vi "local.Reserve.vi"(0 "SLSC Local in":refnum<class "SLSC Interface.lvclass">, 5 "devices":refnum<k21>="$DefaultDevices", 7 "reservation access (Read/Write)":i32(ring)=3 items=["Read Only"=1, "Read/Write"=3], 9 "reservation group":string, 11 "error in (no error)":errorcluster) -> (4 "SLSC Local out":refnum<class "SLSC Interface.lvclass">, 15 "error out":errorcluster)   [LabVIEW 2016, in "SLSC Interface.lvclass"]
uses:
  SLSC Interface Class/SLSC Interface.lvclass
  SLSC Interface Class/Read session.vi
  SLSC Interface Class/Write session.vi
  <vilib>/SLSC/SLSC.lvlib
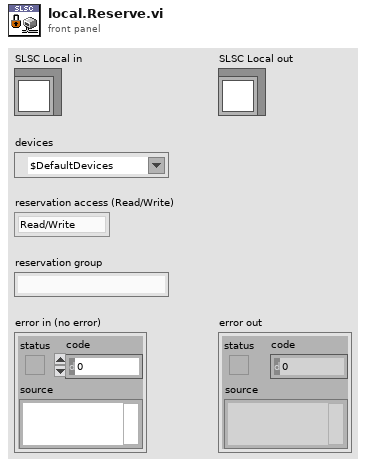
[diagram p1: front panel]
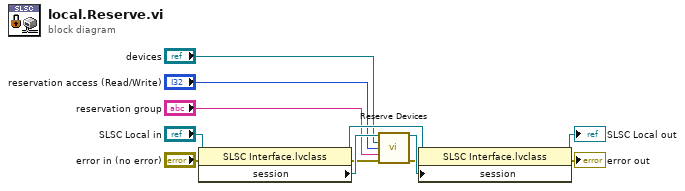
[diagram p0: block diagram]
diagram:
  n1 = property class="SLSC Interface.lvclass"(reference="SLSC Local in", error in="error in (no error)") -> (reference out=w11:refnum<class "SLSC Interface.lvclass">, error out=w8:errorcluster, "session"=w9:refnum<k21>)
  n2 = call <vilib>:"Reserve Devices.vi"("session in"=w9, "devices"="devices", "reservation access (Read/Write)"="reservation access (Read/Write)", "reservation group"="reservation group", "error in (no error)"=w8) -> ("session out"=w7:refnum<k21>, "error out"=w6:errorcluster)  [unwired: 9 in]
  n3 = property class="SLSC Interface.lvclass"(reference=w11, error in=w6, "session"=w7) -> (reference out=→"SLSC Local out":refnum<class "SLSC Interface.lvclass">, error out=→"error out":errorcluster)
